vi "calculatecoefficientjob.vi"(7 "Tangent":T1, 10 "sample sn":string[](array[string]), 11 "sample port":refnum<visa-resource-name>[](array[refnum])) -> (0 "tangent":dbl[][](array[numeric]), 1 "do":dbl[](array[numeric]))   [LabVIEW 2012]
uses:
  globalstatus.vi
  globalreport.vi
panel:
  out "Times":dbl
  in  "Tolerance":dbl
  in  "expect":dbl[](array[numeric])
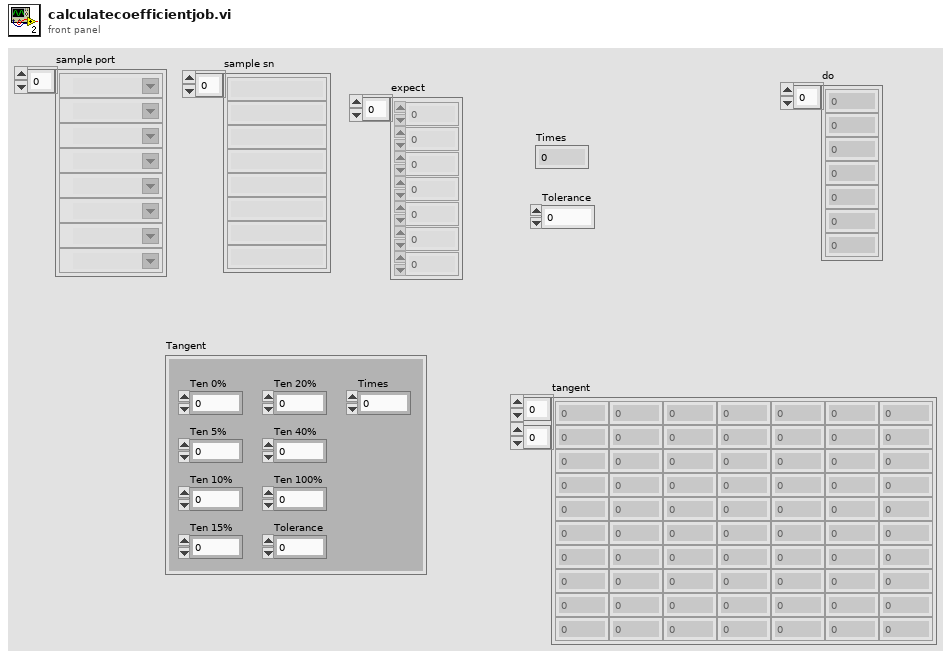
[diagram p1: front panel]
types:
  T1 = cluster{"Ten 0%":dbl, "Ten 5%":dbl, "Ten 10%":dbl, "Ten 20%":dbl, "Tolerance":dbl, "Ten 15%":dbl, "Ten 40%":dbl, "Ten 100%":dbl, "Times":dbl}
  T2 = cluster{"PORT":string, "SN":string, "RED DAC":dbl, "BLUE DAC":dbl, "RED AMP":dbl, "BLUE AMP":dbl, "T0":dbl, "T1":dbl, "T2":dbl, "T3":dbl, "T4":dbl, "T5":dbl, "T6":dbl, "A0":dbl, "A1":dbl, "A2":dbl, "A3":dbl, "B0":dbl, "B1":dbl, "B2":dbl, "C1":dbl, "C0":dbl, "result":string, "error":string}[]
  T3 = cluster{"PORT":string, "SN":string, "RED DAC":dbl, "BLUE DAC":dbl, "RED AMP":dbl, "BLUE AMP":dbl, "T0":dbl, "T1":dbl, "T2":dbl, "T3":dbl, "T4":dbl, "T5":dbl, "T6":dbl, "A0":dbl, "A1":dbl, "A2":dbl, "A3":dbl, "B0":dbl, "B1":dbl, "B2":dbl, "C1":dbl, "C0":dbl, string, string}
  T4 = cluster{"PORT":string, "SN":string, "RED DAC":dbl, "BLUE DAC":dbl, "RED AMP":dbl, "BLUE AMP":dbl, "Numeric":dbl, "Numeric":dbl, "Numeric":dbl, "Numeric":dbl, "Numeric":dbl, "Numeric":dbl, "Numeric":dbl, "A0":dbl, "A1":dbl, "A2":dbl, "A3":dbl, "B0":dbl, "B1":dbl, "B2":dbl, "C1":dbl, "C0":dbl, "result":string, "error":string}
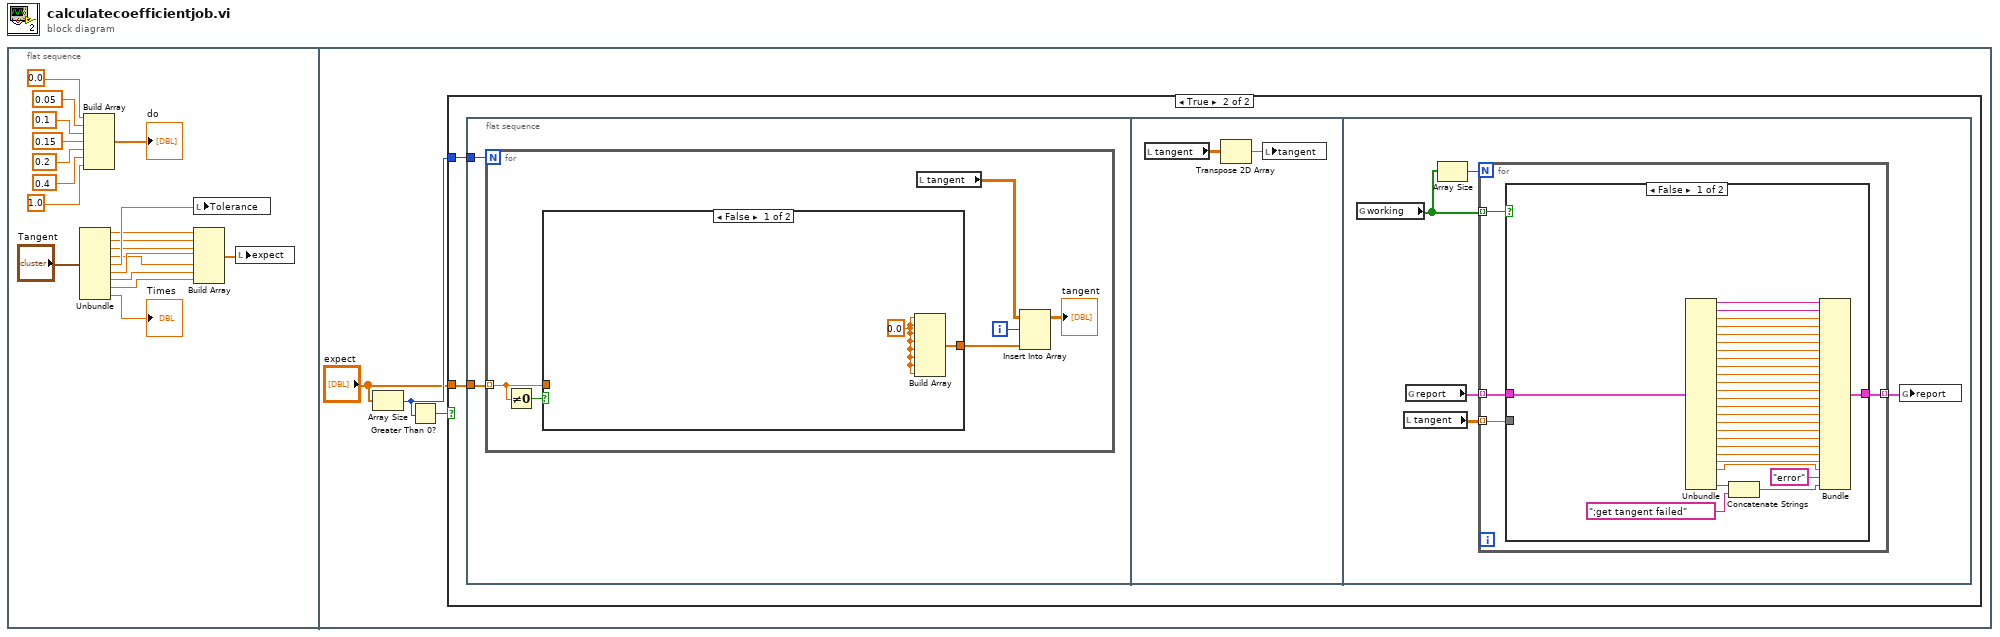
[diagram p0: block diagram]
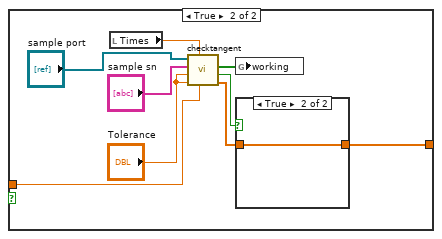
[diagram p3: hidden frame]
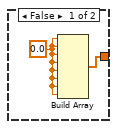
[diagram p4: hidden frame]
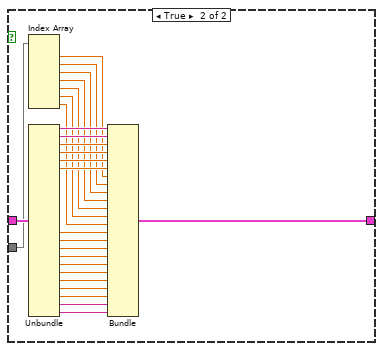
[diagram p5: hidden frame]
diagram:
  n1 = flat-sequence {
    frame #0 {
      n2 = Unbundle("Tangent") -> ("Ten 0%"=w17:dbl, "Ten 5%"=w16:dbl, "Ten 10%"=w15:dbl, "Ten 20%"=w13:dbl, "Tolerance"=w18:dbl, "Ten 15%"=w14:dbl, "Ten 40%"=w12:dbl, "Ten 100%"=w11:dbl, "Times"=→"Times":dbl)
      n3 = Build Array(0.0, 0.05, 0.1, 0.15, 0.2, 0.4, 1.0) -> (→"do":dbl[])
      n4 = local write "Tolerance"(w18) -> ()
      n5 = Build Array(w17, w16, w15, w14, w13, w12, w11) -> (w10:dbl[])
      n6 = local write "expect"(w10) -> ()
    }
    frame #1 {
      n7 = Array Size(array="expect") -> (size(s)=w21:i32)
      n8 = Greater Than 0?(x=w21) -> (x > 0?=w22:bool)
      n9 = case shown="True" w22 {
        tunnel: w21 -> [_ w24]
        tunnel: "expect" -> [_ w23]
        frame False {
        }
        frame True {
          n10 = flat-sequence {
            tunnel: w24 -> [w26]
            tunnel: w23 -> [w25]
            frame #0 {
              n11 = for {
                N: w26 -> [_]
                tunnel: w25 -> [w32] mode=indexing
                i -> [w27]
                n12 = Not Equal To 0?(x=w32) -> (x != 0?=w31:bool)
                n13 = case shown="False" w31 {
                  tunnel: w32 -> [_ w41]
                  tunnel: [w33 w36] -> w30
                  frame False {
                    w34 = 0.0
                    n14 = Build Array(w34, w34, w34, w34, w34, w34, w34, w34) -> (w33:dbl[])
                  }
                  frame True {
                    n15 = local read "Times"() -> (w35:dbl)
                    n16 = call "checktangent.vi"("expect tangent"=w41, "times"=w35, "down"="Tolerance", "up"="Tolerance", "sample sn"="sample sn", "sample port"="sample port") -> ("tangnet"=w37:dbl[], "ok"=w38:bool, "Array"=w39:bool[])  [unwired: 3 in]
                    n17 = global write "globalstatus.vi" "working"(w39) -> ()
                    n18 = case shown="True" w38 {
                      tunnel: w37 -> [_ w46]
                      tunnel: [w44 w46] -> w36
                      frame False {
                        w45 = 0.0
                        n19 = Build Array(w45, w45, w45, w45, w45, w45, w45, w45) -> (w44:dbl[])
                      }
                      frame True {
                      }
                    }
                  }
                }
                n20 = local read "tangent"() -> (w28:dbl[][])
                n21 = Insert Into Array(array=w28, index (row)=w27, new element=w30) -> (→"tangent":dbl[][])  [unwired: 1 in]
              }
            }
            frame #1 {
              n22 = local read "tangent"() -> (w48:dbl[][])
              n23 = Transpose 2D Array(2D array=w48) -> (transposed array=w47:dbl[][])
              n24 = local write "tangent"(w47) -> ()
            }
            frame #2 {
              n25 = global read "globalstatus.vi" "working"() -> (w49:bool[])
              n26 = local read "tangent"() -> (w50:dbl[][])
              n27 = global read "globalreport.vi" "report"() -> (w52:T2)
              n28 = Array Size(array=w49) -> (size(s)=w53:i32)
              n29 = for {
                N: w53 -> [_]
                tunnel: w49 -> [w57] mode=indexing
                tunnel: w52 -> [w56] mode=indexing
                tunnel: [w55] -> w51 mode=indexing
                tunnel: w50 -> [w54] mode=indexing
                n30 = case shown="False" w57 {
                  tunnel: w56 -> [w85 w112]
                  tunnel: [w83 w94] -> w55
                  tunnel: w54 -> [_ w87]
                  frame False {
                    n31 = Unbundle(w85) -> ("PORT"=w84:string, "SN"=w82:string, "RED DAC"=w81:dbl, "BLUE DAC"=w80:dbl, "RED AMP"=w79:dbl, "BLUE AMP"=w78:dbl, "T0"=w77:dbl, "T1"=w76:dbl, "T2"=w75:dbl, "T3"=w74:dbl, "T4"=w73:dbl, "T5"=w72:dbl, "T6"=w71:dbl, "A0"=w70:dbl, "A1"=w69:dbl, "A2"=w68:dbl, "A3"=w67:dbl, "B0"=w66:dbl, "B1"=w65:dbl, "B2"=w64:dbl, "C1"=w63:dbl, "C0"=w62:dbl, "error"=w60:string)  [unwired: 1 out]
                    n32 = Concatenate Strings(w60, ";get tangent failed") -> (w58:string)
                    n33 = Bundle("PORT"=w84, "SN"=w82, "RED DAC"=w81, "BLUE DAC"=w80, "RED AMP"=w79, "BLUE AMP"=w78, "T0"=w77, "T1"=w76, "T2"=w75, "T3"=w74, "T4"=w73, "T5"=w72, "T6"=w71, "A0"=w70, "A1"=w69, "A2"=w68, "A3"=w67, "B0"=w66, "B1"=w65, "B2"=w64, "C1"=w63, "C0"=w62, "error", w58) -> (w83:T3)  [unwired: 1 in]
                  }
                  frame True {
                    n34 = Index Array(array=w87) -> (element #1=w93:dbl, element #2=w92:dbl, element #3=w91:dbl, element #4=w90:dbl, element #5=w89:dbl, element #6=w88:dbl, element #7=w86:dbl)  [unwired: 7 in]
                    n35 = Unbundle(w112) -> ("PORT"=w111:string, "SN"=w110:string, "RED DAC"=w109:dbl, "BLUE DAC"=w108:dbl, "RED AMP"=w107:dbl, "BLUE AMP"=w106:dbl, "A0"=w105:dbl, "A1"=w103:dbl, "A2"=w104:dbl, "A3"=w102:dbl, "B0"=w101:dbl, "B1"=w100:dbl, "B2"=w99:dbl, "C1"=w98:dbl, "C0"=w97:dbl, "result"=w96:string, "error"=w95:string)  [unwired: 7 out]
                    n36 = Bundle("PORT"=w111, "SN"=w110, "RED DAC"=w109, "BLUE DAC"=w108, "RED AMP"=w107, "BLUE AMP"=w106, "Numeric"=w93, "Numeric"=w92, "Numeric"=w91, "Numeric"=w90, "Numeric"=w89, "Numeric"=w88, "Numeric"=w86, "A0"=w105, "A1"=w103, "A2"=w104, "A3"=w102, "B0"=w101, "B1"=w100, "B2"=w99, "C1"=w98, "C0"=w97, "result"=w96, "error"=w95) -> (w94:T4)  [unwired: 1 in]
                  }
                }
              }
              n37 = global write "globalreport.vi" "report"(w51) -> ()
            }
          }
        }
      }
    }
  }
